vi "Path to Drive.vi"(4 "Path":path) -> (7 "Drive":string)   [LabVIEW 2020, in "Volatus.lvlib" / "Windows System SAL.lvclass"]
uses:
  Windows System SAL.lvclass
  Windows System SAL.lvclass/Windows System SAL.ctl
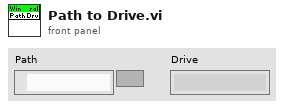
[diagram p1: front panel]
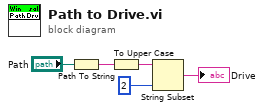
[diagram p0: block diagram]
diagram:
  n1 = Path To String(path="Path") -> (string=w4:string)
  n2 = To Upper Case(1:w4) -> (0:w1:string)
  n3 = String Subset(string=w1, length (rest)=2 ("length (rest)")) -> (substring=→"Drive":string)  [unwired: 1 in]
